vi "20210415_01_ATA_FPGA.vi"() -> ()   [LabVIEW 2018]
doc: "This FPGA VI transfers data samples to the host using a stream. The stream is controlled from the host."
uses:
  <vilib>/Platform/TimedLoop/XDataNode/wakeup.ctl
  <vilib>/Platform/TimedLoop/XDataNode/XDNodeRunTimeDep.lvlib
  <vilib>/Platform/TimedLoop/XDataNode/nitl_modes.ctl
  <vilib>/Platform/TimedLoop/XDataNode/timing_clust.ctl
  <vilib>/Platform/TimedLoop/XDataNode/XDataNode.xnode
  <vilib>/eio/EIONode/EIONode.xnode
  <vilib>/rvi/eio/common/nirviEmuTemplateMethod_errors.vi
  <vilib>/rvi/DataTransferAndStorage/Container/XNode/niFpgaContainer.xnode
  <instrlib>/_niInstr/Basic Elements/v1/FPGA/niInstr Basic Elements v1 FPGA.lvlib
  <vilib>/rvi/FXPMathLib/FxpInterpret/XNode/nifxpmath_Interpret.xnode
  <vilib>/rvi/FXPMathLib/FxpMul/XNode/nifxpmath_Multiplier.xnode
  <vilib>/rvi/FXPMathLib/sim/FxpSim.dll
  <vilib>/rvi/FXPMathLib/FxpAdd/XNode/nifxpmath_Add.xnode
  <vilib>/rvi/Analysis/measure/FFT/XNode/niFpgaFFT.xnode
  <instrlib>/_niInstr/Basic Elements/v1/FPGA/Private/Count Up U32.vi
  <vilib>/rvi/Memory/Memory_Emulation/niFpgaMemoryEmulationRefIn.vi
  <vilib>/fxp/LVFixedPointQuantizationPolicyTypeDef.ctl
  <vilib>/rvi/Analysis/measure/FFT/simModelSupport/niFpgaFFTSimDfxp.ctl
  <vilib>/rvi/Analysis/measure/FFT/simModelSupport/niFpgaFFTSimArithmeticProperties.ctl
  <vilib>/rvi/Analysis/measure/FFT/simModelSupport/niFPGA FFT Sim Types.ctl
  <vilib>/rvi/Analysis/measure/FFT/simModelSupport/niFPGA FFT Outside SCTL Sim Properties.ctl
  <vilib>/rvi/Analysis/measure/FFT/simModelSupport/niFpgaFFTSimModelOutsideSCTLCore.vi
  <vilib>/rvi/LocalResourceManager/LocalResourceManager.xnode
  <vilib>/rvi/DataTransferAndStorage/Container/Common/niFpgaContainerGetUniqueNameForEmu.vi
  <vilib>/rvi/DataTransferAndStorage/Container/Common/niFpgaContainerSetEmuInfo.vi
  <vilib>/rvi/eio/common/nirviEmuReportErrorAndStop.vi
  <vilib>/rvi/FIFO/Fifo_Resource/niFpgaFifoEmulationRefIn.vi
  <vilib>/rvi/FIFO/Fifo_Resource/nirvififoEmulationRead.vi
  <vilib>/rvi/interface/RandomDataEmulation/nirviRandomDataFpgaMultiElementTemplate.vi
  <instrlib>/_niInstr/Basic Elements/v1/FPGA/Private/Count Up U16.vi
  FPGA_Controls/FilterStageEnum.ctl
  FPGA_Controls/FPGA_Enable_Clust.ctl
  FPGA_Controls/FPGA_Shift_Enable.ctl
  <instrlib>/_niInstr/Basic Elements/v1/FPGA/Private/Count Up U8.vi
  FPGA_Controls/FPGA_Scale_Clust.ctl
  FPGA_Controls/FPGA_Probe_Clust.ctl
panel:
  out "5_Seconds_Elapsed":bool
  out "Write to FIFO 2":bool
  out "Write to FIFO":bool
  in  "EnableFIFO":bool
  out "AI0_Unshifted_Index":u32
  out "AI0_Co_Beac_Q_Index":fxp<+/-,24,1>
  out "AI0_Co_I_Index":fxp<+/-,24,1>
  out "MaxMeas":fxp<+/-,24,1>
  in  "Ramp?":bool
  out "AI1_Over":bool
  out "AI0_Over":bool
  in  "Simulate?":bool
  out "Chan1_Beac_QProbe":T1
  out "Chan1_Beac_IProbe":T1
  out "Chan1_Cal_QProbe":T1
  out "Chan0_Beac_QProbe":T1
  out "Chan0_Beac_IProbe":T1
  out "Chan0_Cal_QProbe":T1
  out "NoiseFloorFFT_LoopCount 2":i32
  out "ReceiverTimed Out 2":bool
  out "SuccessiveIndeces 2":u16[](array[numeric])
  in  "#Avg 2":u16=1
  in  "ScaleMeasurement 2":fxp<+/-,16,1>
  in  "Scale_Step1_2":fxp<+/-,17,17>
  in  "EnableStep1_2":bool
  out "Probe 2_2":fxp<+/-,16,16>
  out "Probe 3_2":fxp<+/-,16,1>
  out "Probe 5_2":fxp<+/-,16,2>
  out "Probe 7_2":fxp<+/-,18,1>
  in  "Scale_NoiseFloor 2":fxp<+/-,30,30>
  out "Probe 21_2":fxp<+/-,24,5>
  out "Probe 22_2":fxp<+/-,54,35>
  out "Probe 23_2":fxp<+/-,54,1>
  out "Probe 24_2":fxp<+/-,16,1>
  in  "Offset 2":fxp<+/-,16,16>
  in  "Scale 2":T2={"Scale_Step4"=1.0, "Scale_Step5"=1.0, "Scale_Step6"=1.0, "Scale_Step7"=1.0}
  in  "Enable 2":T3
  in  "FreqShiftCal 2":fxp<+/-,48,0> format="%#.48g"
  out "Chan1_Cal_IProbe":T1
  in  "FreqShiftBeac 2":fxp<+/-,48,0> format="%#.48g"
  out "NoiseFloorFIFOTimeOut 2":bool
  out "Sends 2":u32
  in  "SampleCountReset 2":u32=125000000
  out "Probe 1_2":i16
  out "Probe Offsetd 2":fxp<+/-,16,16>
  out "Probe Offsetd":fxp<+/-,16,16>
  in  "Sample Clock Commit":bool
  in  "Sample Clock Select":u8
  out "SPI Idle":bool
  out "Configuration Error":bool
  out "Synthesizer Locked":bool
  out "Probe 1":i16
  in  "#Avg":u16=1
  in  "SampleCountReset":u32=125000000
  out "ReceiverTimed Out":bool
  out "Sends":u32
  out "SuccessiveIndeces":u16[](array[numeric])
  out "NoiseFloorFFT_LoopCount":i32
  out "NoiseFloorFIFOTimeOut":bool
  in  "FreqShiftBeac":fxp<+/-,48,0> format="%#.48g"
  out "AI0_Cal_IProbe":T1
  in  "Scale":T2={"Scale_Step4"=1.0, "Scale_Step5"=1.0, "Scale_Step6"=1.0, "Scale_Step7"=1.0}
  in  "Enable":T3
  in  "Offset":fxp<+/-,16,16>
  out "Probe 24":fxp<+/-,16,1>
  out "Probe 23":fxp<+/-,54,1>
  out "Probe 22":fxp<+/-,54,35>
  out "Probe 21":fxp<+/-,24,5>
  in  "Scale_NoiseFloor":fxp<+/-,30,30>
  out "Probe 7":fxp<+/-,18,1>
  out "Probe 5":fxp<+/-,16,2>
  out "Probe 3":fxp<+/-,16,1>
  out "Probe 2":fxp<+/-,16,16>
  in  "EnableStep1":bool
  in  "Scale_Step1":fxp<+/-,17,17>
  in  "ScaleMeasurement":fxp<+/-,16,1>
  in  "FreqShiftCal":fxp<+/-,48,0> format="%#.48g"
  out "IO Module\\Initialization Done":bool
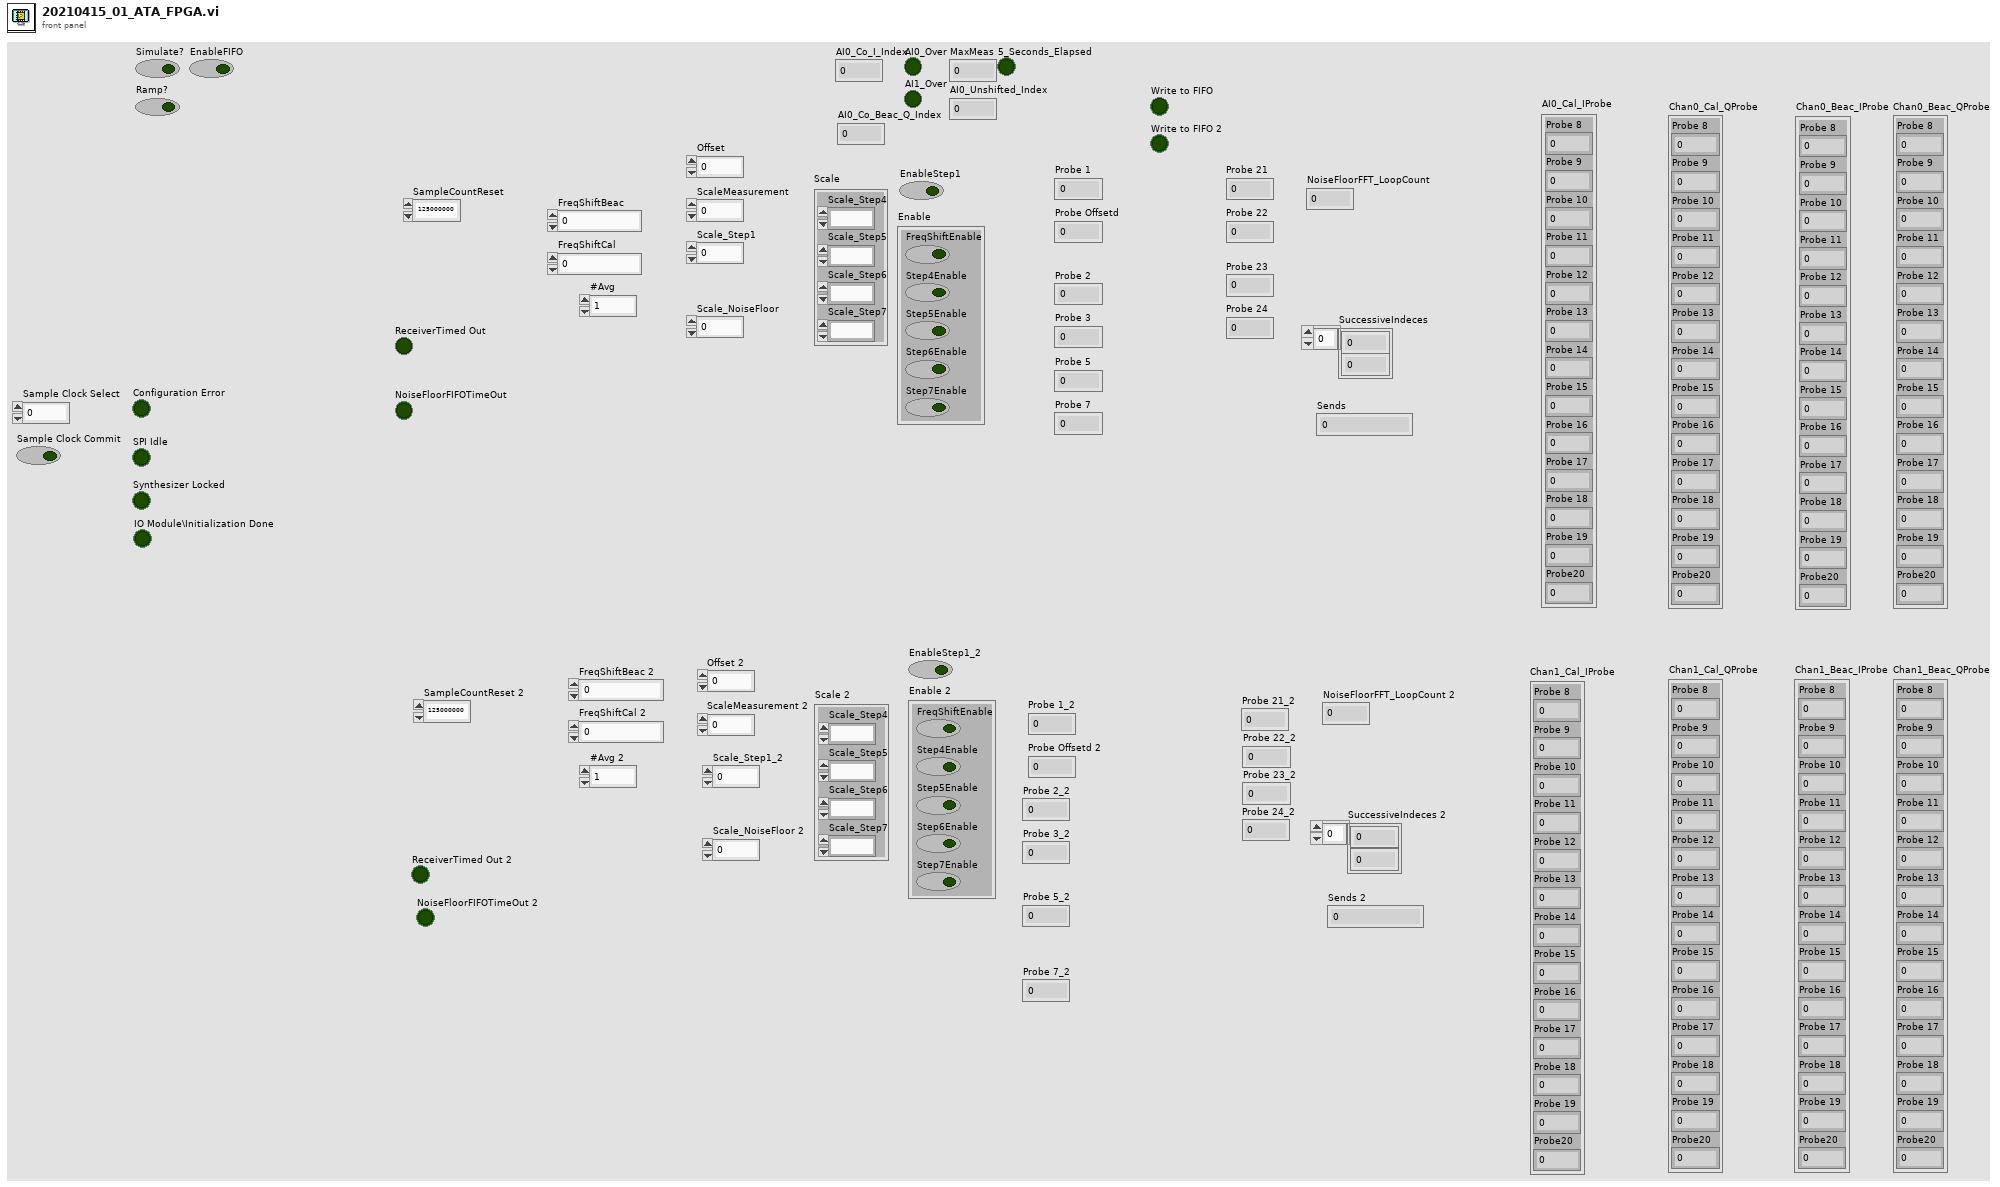
[diagram p1: front panel]
types:
  T1 = typedef "FPGA_Probe_Clust.ctl" = cluster{"Probe 8":fxp<+/-,18,1>, "Probe 9":fxp<+/-,24,1>, "Probe 10":fxp<+/-,24,1>, "Probe 11":fxp<+/-,24,1>, "Probe 12":fxp<+/-,47,24>, "Probe 13":fxp<+/-,24,1>, "Probe 14":fxp<+/-,25,2>, "Probe 15":fxp<+/-,48,25>, "Probe 16":fxp<+/-,24,1>, "Probe 17":fxp<+/-,25,2>, "Probe 18":fxp<+/-,48,25>, "Probe 19":fxp<+/-,24,1>, "Probe20":fxp<+/-,24,1>}
  T2 = typedef "FPGA_Scale_Clust.ctl" = cluster{"Scale_Step4":fxp<+/-,23,23>, "Scale_Step5":fxp<+/-,23,23>, "Scale_Step6":fxp<+/-,23,23>, "Scale_Step7":fxp<+/-,23,23>}
  T3 = typedef "FPGA_Enable_Clust.ctl" = cluster{"FreqShiftEnable":bool, "Step4Enable":bool, "Step5Enable":bool, "Step6Enable":bool, "Step7Enable":bool}
  T4 = typedef "XDNodeRunTimeDep.lvlib/timing_clust.ctl" = cluster{"Expected End [f-1]":u64, "Actual End [f-1]":u64, "Finished Late? [f-1]":bool, "Expected End [i-1]":u64, "Actual End [i-1]":u64, "Finished Late? [i-1]":bool, "Expected Start [i]":u64, "Actual Start [i]":u64, "Expected Start [f]":u64, "Actual Start [f]":u64, "Source Name":string, "Structure Name":string, "Period":i64, "Deadline":i64, "Offset":i64, "Start":i64, "Priority":i32, "Timeout":i32, "Mode":T5, "Wakeup Reason":T6, "Error":errorcluster, "Source Type":string, "Secondary Source Type":string, "Global End Time":u64, "Global Start Time":u64, "Frame Duration":u64, "Iteration Duration":u64, "Assigned CPU":i32, "I/O Scan Engine Mode":u32}
  T5 = typedef "XDNodeRunTimeDep.lvlib/nitl_modes.ctl" = enum32{"No Change", "Process missed periods, maintain original phase", "Discard missed periods, maintain original phase", "Process missed periods, ignore original phase", "Discard missed periods, ignore original phase"}
  T6 = typedef "XDNodeRunTimeDep.lvlib/wakeup.ctl" = enum32{"Normal", "Aborted", "Asynchronous wakeup", "Timing source error", "Timed loop error", "Timeout"}
  T7 = typedef "FPGA_Shift_Enable.ctl" = cluster{"EnableFIFO":bool, "EnableStages":T3}
  T8 = typedef "FilterStageEnum.ctl" = enum16{"Digitiz0", "Digitiz1", "ScaleMeas", "Scale1", "Scale4", "Scale5", "Scale6", "Scale7"}
  T9 = typedef "FPGA_ShiftOutput.ctl" = cluster{"Index":fxp<+/-,24,1>, "output valid":bool, "Data out":fxp<+/-,24,1>, "Probe":T1}
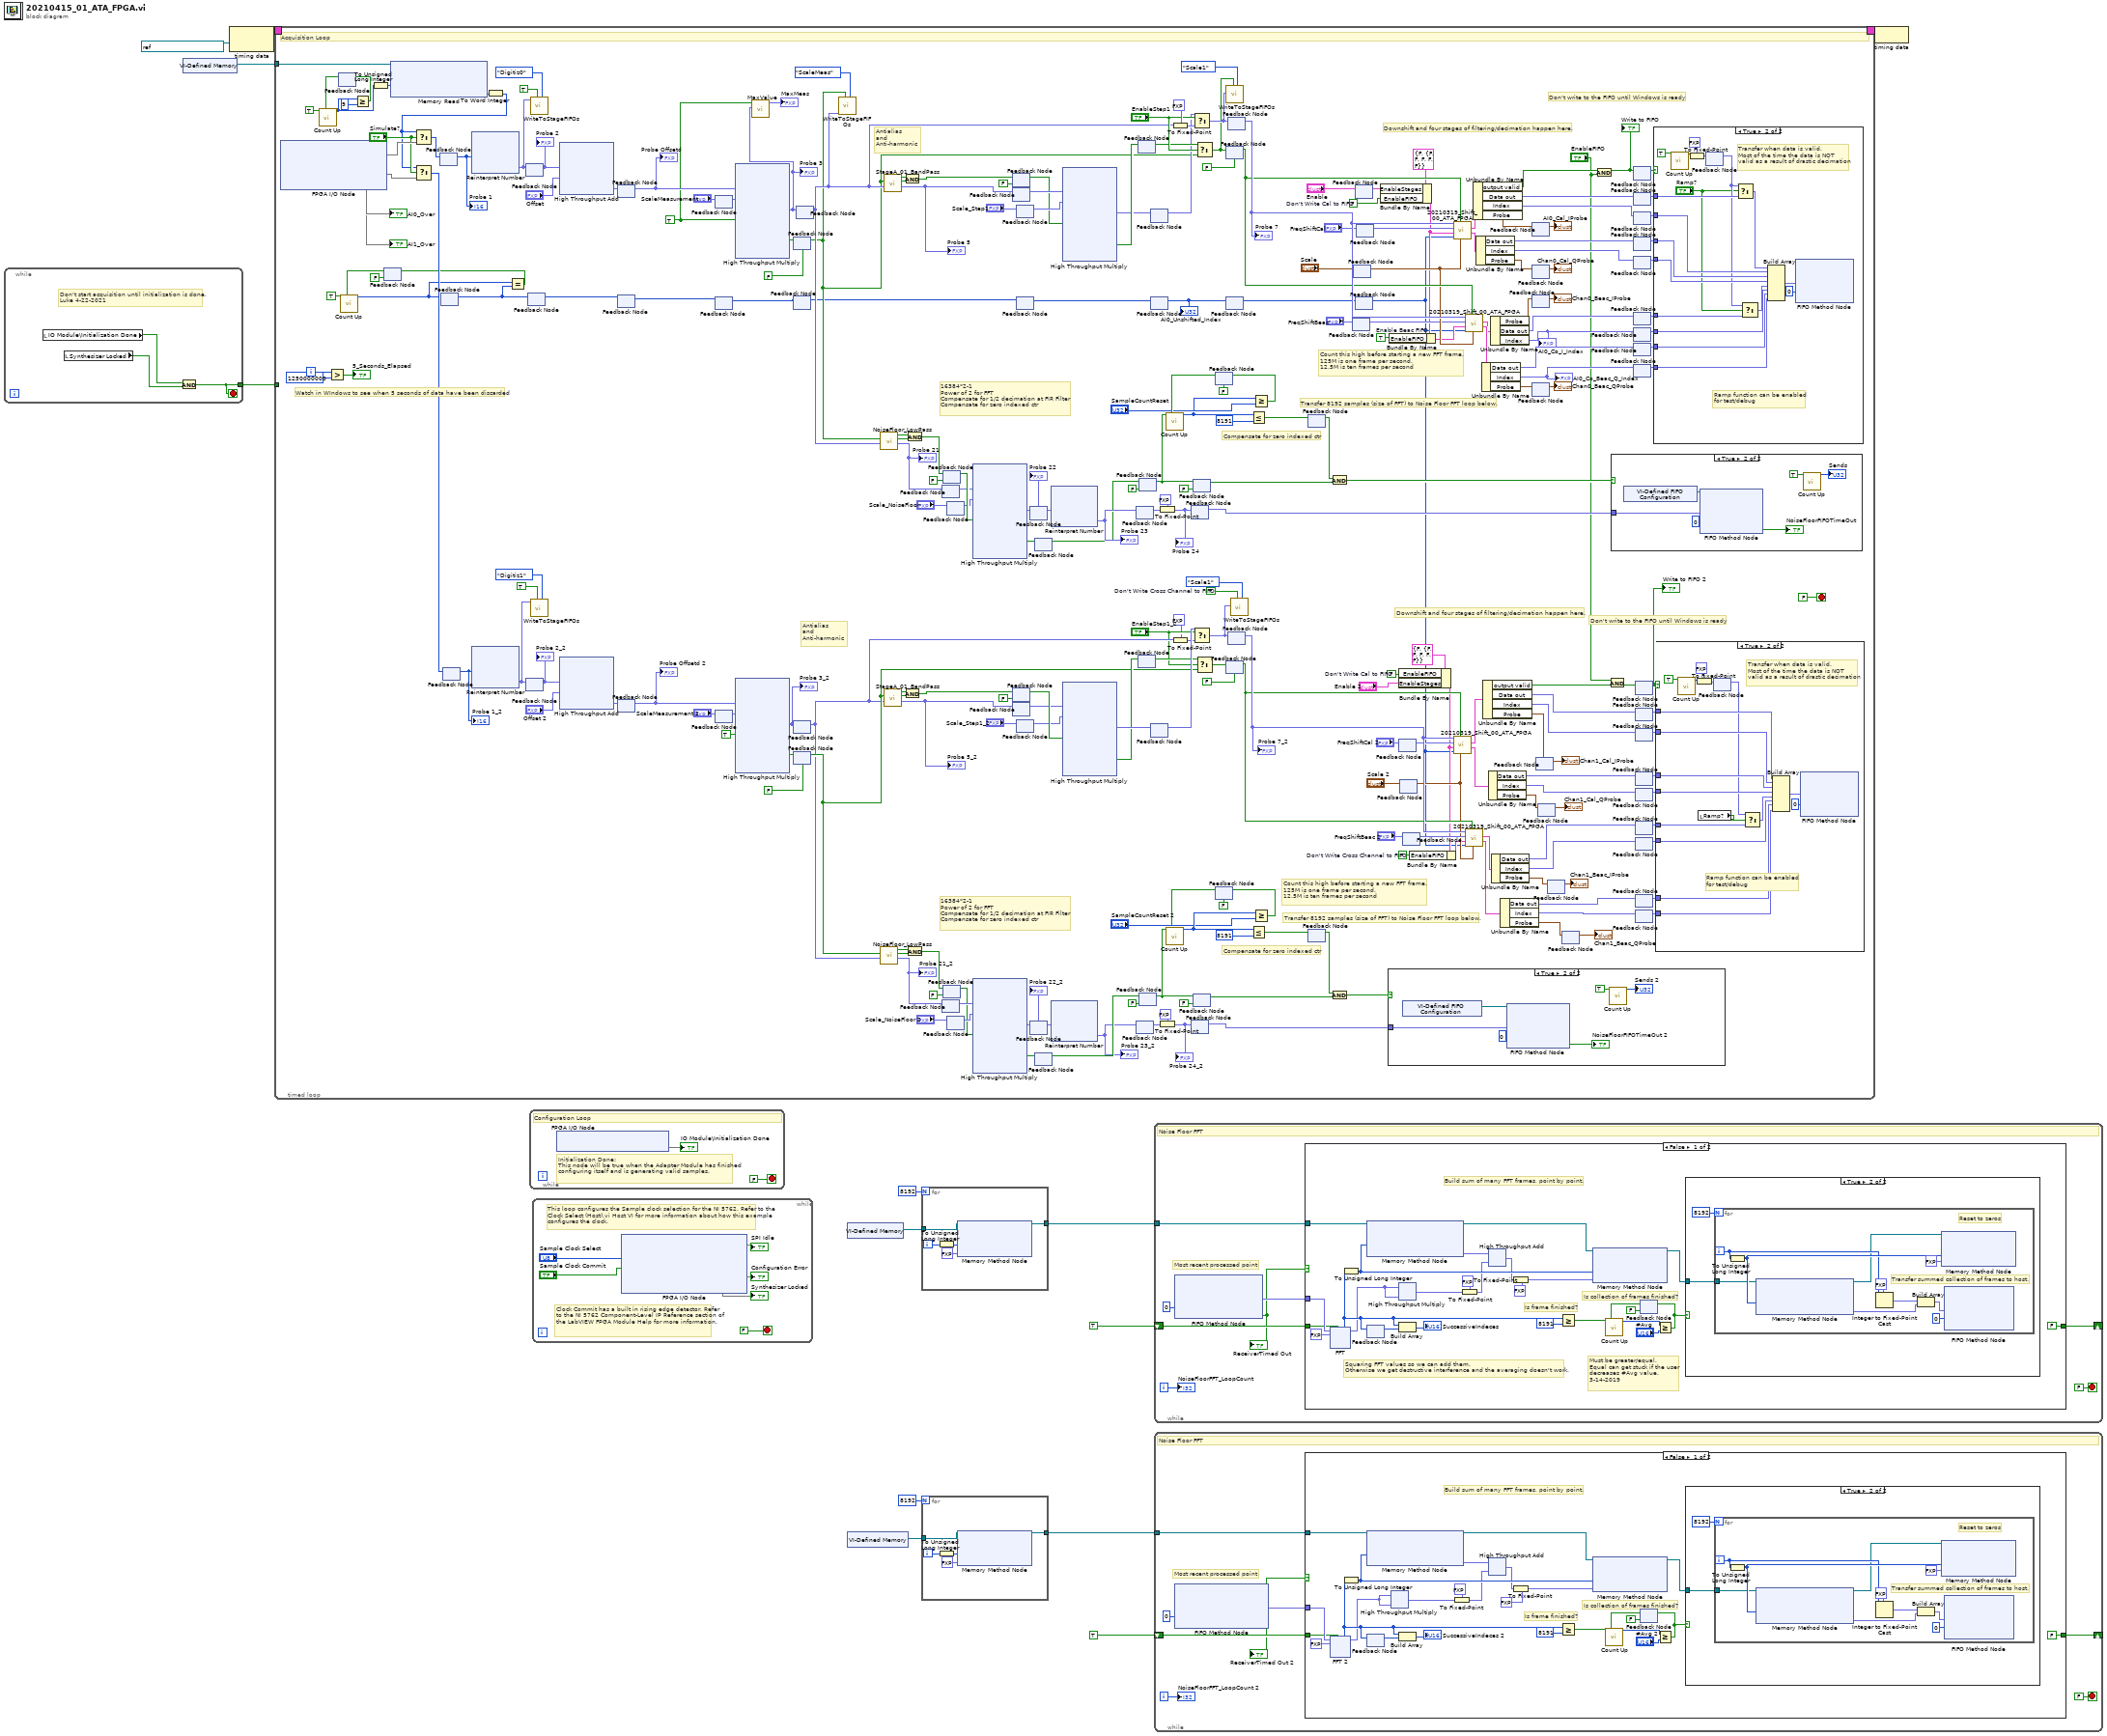
[diagram p0: block diagram]
diagram:
  n1 = while {
    tunnel: [w14] -> w1
    stop <- w14 stop-if-true
    # "Don't start acquisition until initialization is done.\nLuke 4-22-2021"
    n2 = local read "IO Module\\Initialization Done"() -> (w16:bool)
    n3 = local read "Synthesizer Locked"() -> (w15:bool)
    n4 = And(x=w16, y=w15) -> (x .and. y?=w14:bool)
  }
  n5 = xnode "VI-Defined Memory"() -> ("Memory Out"=w2:refnum<k21>)
  n6 = node-c288(refnum<k21> "IO Module\\Data Clock" ("Source Name")) -> (w13:T4)
  n7 = timed-loop {
    timing: w13 -> [_]
    timing-out: [_] -> w12
    tunnel: w2 -> [w118]
    tunnel: w1 -> [_]
    i -> [w19]
    stop <- FALSE stop-if-true
    w66 = FALSE  # Don't Write Cal to FIFO
    w63 = TRUE  # Enable Beac FIFO
    w94 = FALSE  # Don't Write Cross Channel to FIFO
    w52 = FALSE  # Don't Write Cross Channel to FIFO
    w58 = FALSE  # Don't Write Cal to FIFO
    w107 = TRUE ("input valid")
    # "Watch in WIndows to see when 5 seconds of data have been discarded"
    # "Don't write to the FIFO until Windows is ready"
    # "Don't write to the FIFO until Windows is ready"
    # "Downshift and four stages of filtering/decimation happen here."
    # "Downshift and four stages of filtering/decimation happen here."
    # "Antialias\nand\nAnti-harmonic"
    # "Compensate for zero indexed ctr"
    # "16384*2-1\nPower of 2 for FFT\nCompensate for 1/2 decimation at FIR Filter\nCompensate for zero indexed ctr"
    # "Transfer 8192 samples (size of FFT) to Noise Floor FFT loop below."
    # "Count this high before starting a new FFT frame.\n125M is one frame per second.\n12.5M is ten frames per second"
    # "Antialias\nand\nAnti-harmonic"
    # "Compensate for zero indexed ctr"
    # "16384*2-1\nPower of 2 for FFT\nCompensate for 1/2 decimation at FIR Filter\nCompensate for zero indexed ctr"
    # "Transfer 8192 samples (size of FFT) to Noise Floor FFT loop below."
    # "Count this high before starting a new FFT frame.\n125M is one frame per second.\n12.5M is ten frames per second"
    # "Acquisition Loop"
    n8 = xnode "FPGA I/O Node"() -> ("IO Module\\AI 0 Data"=w117, "IO Module\\AI 0 Over Range"=→"AI0_Over", "IO Module\\AI 1 Data"=w112, "IO Module\\AI 1 Over Range"=→"AI1_Over")  [unwired: 4 in, 4 out]
    n9 = Greater?(x=w19, y=1250000000) -> (0:→"5_Seconds_Elapsed":bool)
    n10 = feedback #1() -> (w119:bool)  [unwired: 1 in]
    n11 = call-poly <instrlib>:"Count Up.vi"("increment"=TRUE, "reset"=w119) -> ("count out"=w122:u8)  [unwired: 13 in]
    n12 = Greater Or Equal?(x=w122, y=u8 9) -> (x >= y?=w120:bool)
    n13 = feedback-in #1(w120) -> ()
    n14 = To Unsigned Long Integer(number=w122) -> (unsigned 32bit integer=w124:u32)
    n15 = feedback #2(FALSE) -> (w28:bool)
    n16 = call-poly <instrlib>:"Count Up.vi"("increment"=TRUE, "reset"=w28) -> ("count out"=w26:u32)  [unwired: 13 in]
    n17 = xnode ("Memory Read")("Address"=w124, "Memory In"=w118) -> ("Data"=w115:i8)  [unwired: 1 out]
    n18 = feedback #3() -> (w226:i16)  [unwired: 1 in]
    "Probe 1" <- w226
    n19 = feedback #4() -> (w25:u32)  [unwired: 1 in]
    n20 = feedback-in #4(w26) -> ()
    n21 = feedback #5() -> (w207:i16)  [unwired: 1 in]
    "Probe 1_2" <- w207
    n22 = xnode "Reinterpret Number"("x"=w226) -> ("y"=w98:fxp<+/-,16,16>)
    n23 = xnode "Reinterpret Number"("x"=w207) -> ("y"=w97:fxp<+/-,16,16>)
    n24 = To Word Integer(number=w115) -> (16bit integer=w111:i16)
    n25 = Select(t=w111, s="Simulate?", f=w117) -> (s? t:f=w116:i16)
    n26 = Select(t=w111, s="Simulate?", f=w112) -> (s? t:f=w113:i16)
    n27 = feedback-in #3(w116) -> ()
    n28 = feedback-in #5(w113) -> ()
    n29 = Equal?(x=w26, y=w25) -> (x = y?=w29:bool)
    n30 = feedback-in #2(w29) -> ()
    n31 = feedback #6() -> (w239:fxp<+/-,16,16>)  [unwired: 1 in]
    "Probe 2" <- w239
    n32 = feedback-in #6(w98) -> ()
    n33 = feedback #7() -> (w198:fxp<+/-,16,16>)  [unwired: 1 in]
    "Probe 2_2" <- w198
    n34 = feedback-in #7(w97) -> ()
    n35 = feedback #8() -> (w30:u32)  [unwired: 1 in]
    n36 = feedback-in #8(w25) -> ()
    n37 = call "WriteToStageFIFOs.vi"("Stage"=FilterStageEnum."Digitiz0", "Enable"=TRUE, "Digitiz"=w98) -> ()  [unwired: 9 in]
    n38 = call "WriteToStageFIFOs.vi"("Stage"=FilterStageEnum."Digitiz1", "Enable"=TRUE, "Digitiz"=w97) -> ()  [unwired: 9 in]
    n39 = xnode ("High Throughput Add")("x"=w239, "y"="Offset") -> ("x+y"=w238:fxp<+/-,16,16>)
    n40 = xnode ("High Throughput Add")("x"=w198, "y"="Offset 2") -> ("x+y"=w100:fxp<+/-,16,16>)
    n41 = feedback #9() -> (w108:fxp<+/-,16,16>)  [unwired: 1 in]
    "Probe Offsetd" <- w108
    n42 = feedback-in #9(w238) -> ()
    n43 = feedback #10() -> (w87:u32)  [unwired: 1 in]
    n44 = feedback-in #10(w30) -> ()
    n45 = feedback #11() -> (w99:fxp<+/-,16,16>)  [unwired: 1 in]
    "Probe Offsetd 2" <- w99
    n46 = feedback-in #11(w100) -> ()
    n47 = feedback #12() -> (w267:fxp<+/-,16,1>)  [unwired: 1 in]
    n48 = feedback-in #12("ScaleMeasurement") -> ()
    n49 = feedback #13() -> (w86:u32)  [unwired: 1 in]
    n50 = feedback-in #13(w87) -> ()
    n51 = feedback #14() -> (w168:fxp<+/-,16,1>)  [unwired: 1 in]
    n52 = feedback-in #14("ScaleMeasurement 2") -> ()
    n53 = xnode ("High Throughput Multiply")("x"=w108, "y"=w267, "input valid"=w107) -> ("x*y"=w106:fxp<+/-,16,1>, "output valid"=w241:bool)  [unwired: 1 in, 1 out]
    "Probe 3" <- w106
    n54 = xnode ("High Throughput Multiply")("x"=w99, "y"=w168, "input valid"=TRUE) -> ("x*y"=w165:fxp<+/-,16,1>, "output valid"=w196:bool)  [unwired: 1 in, 1 out]
    "Probe 3_2" <- w165
    n55 = call "MaxValue.vi"("NewValue"=w106, "DataValid"=w107) -> ("Max"=→"MaxMeas":fxp<+/-,24,1>)  [unwired: 9 in]
    n56 = feedback #15(FALSE ("output valid")) -> (w89:bool)
    n57 = feedback-in #15(w241) -> ()
    n58 = feedback #16() -> (w85:u32)  [unwired: 1 in]
    n59 = feedback-in #16(w86) -> ()
    n60 = feedback #17() -> (w210:fxp<+/-,16,1>)  [unwired: 1 in]
    n61 = feedback-in #17(w165) -> ()
    n62 = feedback #18(FALSE ("output valid")) -> (w212:bool)
    n63 = feedback-in #18(w196) -> ()
    n64 = feedback #19() -> (w90:fxp<+/-,16,1>)  [unwired: 1 in]
    n65 = feedback-in #19(w106) -> ()
    n66 = call "WriteToStageFIFOs.vi"("Stage"=FilterStageEnum."ScaleMeas", "Enable"=w89, "ScaleMeas"=w90) -> ()  [unwired: 9 in]
    n67 = call "NoiseFloor_LowPass.vi"("s_axis_data_tdata"=w90, "s_axis_data_tvalid"=w89) -> ("m_axis_data_tdata"=w251:fxp<+/-,24,5>, "m_axis_data_tvalid"=w258:bool, "s_axis_data_tready"=w259:bool)  [unwired: 7 in]
    "Probe 21" <- w251
    n68 = call "NoiseFloor_LowPass.vi"("s_axis_data_tdata"=w210, "s_axis_data_tvalid"=w212) -> ("m_axis_data_tdata"=w186:fxp<+/-,24,5>, "m_axis_data_tvalid"=w179:bool, "s_axis_data_tready"=w178:bool)  [unwired: 7 in]
    "Probe 21_2" <- w186
    n69 = call "StageA_01_BandPass.vi"("s_axis_data_tdata"=w90, "s_axis_data_tvalid"=w89) -> ("m_axis_data_tdata"=w223:fxp<+/-,16,2>, "m_axis_data_tvalid"=w272:bool, "s_axis_data_tready"=w273:bool)  [unwired: 7 in]
    "Probe 5" <- w223
    n70 = call "StageA_01_BandPass.vi"("s_axis_data_tdata"=w210, "s_axis_data_tvalid"=w212) -> ("m_axis_data_tdata"=w211:fxp<+/-,16,2>, "m_axis_data_tvalid"=w162:bool, "s_axis_data_tready"=w161:bool)  [unwired: 7 in]
    "Probe 5_2" <- w211
    n71 = And(x=w273, y=w272) -> (x .and. y?=w224:bool)
    n72 = And(x=w161, y=w162) -> (x .and. y?=w209:bool)
    n73 = And(x=w259, y=w258) -> (x .and. y?=w250:bool)
    n74 = And(x=w178, y=w179) -> (x .and. y?=w187:bool)
    n75 = feedback #20() -> (w252:fxp<+/-,24,5>)  [unwired: 1 in]
    n76 = feedback-in #20(w251) -> ()
    n77 = feedback #21() -> (w185:fxp<+/-,24,5>)  [unwired: 1 in]
    n78 = feedback-in #21(w186) -> ()
    n79 = feedback #22(FALSE ("s_axis_data_tvalid")) -> (w255:bool)
    n80 = feedback-in #22(w250) -> ()
    n81 = feedback #23(FALSE ("s_axis_data_tvalid")) -> (w182:bool)
    n82 = feedback-in #23(w187) -> ()
    n83 = feedback #24() -> (w254:fxp<+/-,30,30>)  [unwired: 1 in]
    n84 = feedback-in #24("Scale_NoiseFloor") -> ()
    n85 = feedback #25() -> (w183:fxp<+/-,30,30>)  [unwired: 1 in]
    n86 = feedback-in #25("Scale_NoiseFloor 2") -> ()
    n87 = xnode ("High Throughput Multiply")("x"=w252, "y"=w254, "input valid"=w255) -> ("x*y"=w247:fxp<+/-,54,35>, "output valid"=w244:bool)  [unwired: 1 in, 1 out]
    "Probe 22" <- w247
    n88 = xnode ("High Throughput Multiply")("x"=w185, "y"=w183, "input valid"=w182) -> ("x*y"=w190:fxp<+/-,54,35>, "output valid"=w193:bool)  [unwired: 1 in, 1 out]
    "Probe 22_2" <- w190
    n89 = feedback #26() -> (w269:fxp<+/-,16,2>)  [unwired: 1 in]
    n90 = feedback-in #26(w223) -> ()
    n91 = feedback #27() -> (w166:fxp<+/-,16,2>)  [unwired: 1 in]
    n92 = feedback-in #27(w211) -> ()
    n93 = feedback #28(FALSE ("s_axis_data_tvalid")) -> (w265:bool)
    n94 = feedback-in #28(w224) -> ()
    n95 = feedback #29(FALSE ("s_axis_data_tvalid")) -> (w170:bool)
    n96 = feedback-in #29(w209) -> ()
    n97 = feedback #30() -> (w266:fxp<+/-,17,17>)  [unwired: 1 in]
    n98 = feedback-in #30("Scale_Step1") -> ()
    n99 = feedback #31() -> (w84:u32)  [unwired: 1 in]
    n100 = feedback-in #31(w85) -> ()
    n101 = feedback #32() -> (w169:fxp<+/-,17,17>)  [unwired: 1 in]
    n102 = feedback-in #32("Scale_Step1_2") -> ()
    n103 = feedback #33() -> (w246:fxp<+/-,54,35>)  [unwired: 1 in]
    n104 = feedback-in #33(w247) -> ()
    n105 = feedback #34() -> (w191:fxp<+/-,54,35>)  [unwired: 1 in]
    n106 = feedback-in #34(w190) -> ()
    n107 = feedback #35() -> (w243:bool)  [unwired: 1 in]
    n108 = feedback-in #35(w244) -> ()
    n109 = feedback #36() -> (w194:bool)  [unwired: 1 in]
    n110 = feedback-in #36(w193) -> ()
    n111 = xnode "Reinterpret Number"("x"=w246) -> ("y"=w245:fxp<+/-,54,1>)
    "Probe 23" <- w245
    n112 = xnode "Reinterpret Number"("x"=w191) -> ("y"=w192:fxp<+/-,54,1>)
    "Probe 23_2" <- w192
    n113 = xnode ("High Throughput Multiply")("x"=w269, "y"=w266, "input valid"=w265) -> ("x*y"=w220:fxp<+/-,18,1>, "output valid"=w222:bool)  [unwired: 1 in, 1 out]
    n114 = xnode ("High Throughput Multiply")("x"=w166, "y"=w169, "input valid"=w170) -> ("x*y"=w215:fxp<+/-,18,1>, "output valid"=w213:bool)  [unwired: 1 in, 1 out]
    n115 = feedback #37() -> (w248:fxp<+/-,54,1>)  [unwired: 1 in]
    n116 = feedback-in #37(w245) -> ()
    n117 = feedback #38() -> (w189:fxp<+/-,54,1>)  [unwired: 1 in]
    n118 = feedback-in #38(w192) -> ()
    n119 = feedback #39() -> (w221:bool)  [unwired: 1 in]
    n120 = feedback-in #39(w222) -> ()
    n121 = feedback #40() -> (w214:bool)  [unwired: 1 in]
    n122 = feedback-in #40(w213) -> ()
    n123 = feedback #41(FALSE ("output valid")) -> (w237:bool)
    n124 = feedback-in #41(w243) -> ()
    n125 = feedback #42(FALSE ("output valid")) -> (w199:bool)
    n126 = feedback-in #42(w194) -> ()
    n127 = feedback #43() -> (w219:fxp<+/-,18,1>)  [unwired: 1 in]
    n128 = feedback-in #43(w220) -> ()
    n129 = feedback #44() -> (w83:u32)  [unwired: 1 in]
    "AI0_Unshifted_Index" <- w83
    n130 = feedback-in #44(w84) -> ()
    n131 = feedback #45() -> (w216:fxp<+/-,18,1>)  [unwired: 1 in]
    n132 = feedback-in #45(w215) -> ()
    n133 = To Fixed-Point(fixed-point type=fxp<+/-,16,1> 0.0, number=w248) -> (fixed-point=w227:fxp<+/-,16,1>)
    "Probe 24" <- w227
    n134 = To Fixed-Point(fixed-point type=fxp<+/-,16,1> 0.0, number=w189) -> (fixed-point=w206:fxp<+/-,16,1>)
    "Probe 24_2" <- w206
    n135 = To Fixed-Point(fixed-point type=fxp<+/-,18,1> 0.0, number=w90) -> (fixed-point=w263:fxp<+/-,18,1>)
    n136 = To Fixed-Point(fixed-point type=fxp<+/-,18,1> 0.0, number=w210) -> (fixed-point=w173:fxp<+/-,18,1>)
    n137 = feedback #46() -> (w228:fxp<+/-,16,1>)  [unwired: 1 in]
    n138 = feedback-in #46(w227) -> ()
    n139 = feedback #47() -> (w205:fxp<+/-,16,1>)  [unwired: 1 in]
    n140 = feedback-in #47(w206) -> ()
    n141 = feedback #48(FALSE ("output valid")) -> (w235:bool)
    n142 = feedback-in #48(w237) -> ()
    n143 = feedback #49(FALSE ("output valid")) -> (w201:bool)
    n144 = feedback-in #49(w199) -> ()
    n145 = Select(t=w219, s="EnableStep1", f=w263) -> (s? t:f=w102:fxp<+/-,18,1>)
    n146 = Select(t=w216, s="EnableStep1_2", f=w173) -> (s? t:f=w95:fxp<+/-,18,1>)
    n147 = Select(t=w221, s="EnableStep1", f=w89) -> (s? t:f=w88:bool)
    n148 = Select(t=w214, s="EnableStep1_2", f=w212) -> (s? t:f=w171:bool)
    n149 = feedback #50(FALSE ("reset")) -> (w278:bool)
    n150 = call-poly <instrlib>:"Count Up.vi"("increment"=w237, "reset"=w278) -> ("count out"=w271:u32)  [unwired: 13 in]
    n151 = feedback #51(FALSE ("reset")) -> (w156:bool)
    n152 = call-poly <instrlib>:"Count Up.vi"("increment"=w199, "reset"=w156) -> ("count out"=w163:u32)  [unwired: 13 in]
    n153 = feedback #52(FALSE ("s_axis_data_tvalid")) -> (w154:bool)
    n154 = feedback-in #52(w88) -> ()
    n155 = feedback #53() -> (w82:u32)  [unwired: 1 in]
    n156 = feedback-in #53(w83) -> ()
    n157 = feedback #54(FALSE ("s_axis_data_tvalid")) -> (w148:bool)
    n158 = feedback-in #54(w171) -> ()
    n159 = call "WriteToStageFIFOs.vi"("Stage"=FilterStageEnum."Scale1", "Enable"=w88, "Scale1"=w102) -> ()  [unwired: 9 in]
    n160 = feedback #55() -> (w218:fxp<+/-,18,1>)  [unwired: 1 in]
    "Probe 7" <- w218
    n161 = feedback-in #55(w102) -> ()
    n162 = feedback #56() -> (w217:fxp<+/-,18,1>)  [unwired: 1 in]
    "Probe 7_2" <- w217
    n163 = feedback-in #56(w95) -> ()
    n164 = call "WriteToStageFIFOs.vi"("Stage"=FilterStageEnum."Scale1", "Enable"=w94, "Scale1"=w95) -> ()  [unwired: 9 in]
    n165 = Less Or Equal?(x=w271, y=u32 8191) -> (x <= y?=w279:bool)
    n166 = Less Or Equal?(x=w163, y=u32 8191) -> (x <= y?=w155:bool)
    n167 = Greater Or Equal?(x=w271, y="SampleCountReset") -> (x >= y?=w275:bool)
    n168 = feedback-in #50(w275) -> ()
    n169 = Greater Or Equal?(x=w163, y="SampleCountReset 2") -> (x >= y?=w159:bool)
    n170 = feedback-in #51(w159) -> ()
    n171 = feedback #57() -> (w236:bool)  [unwired: 1 in]
    n172 = feedback-in #57(w279) -> ()
    n173 = feedback #58() -> (w200:bool)  [unwired: 1 in]
    n174 = feedback-in #58(w155) -> ()
    n175 = And(x=w236, y=w235) -> (x .and. y?=w234:bool)
    n176 = And(x=w200, y=w201) -> (x .and. y?=w202:bool)
    n177 = feedback #59() -> (w137:fxp<+/-,48,0>)  [unwired: 1 in]
    n178 = feedback-in #59("FreqShiftBeac") -> ()
    n179 = feedback #60() -> (w139:T2)  [unwired: 1 in]
    n180 = feedback-in #60("Scale") -> ()
    n181 = feedback #61() -> (w67:T3)  [unwired: 1 in]
    n182 = feedback-in #61("Enable") -> ()
    n183 = feedback #62() -> (w24:u32)  [unwired: 1 in]
    n184 = feedback-in #62(w82) -> ()
    n185 = feedback #63() -> (w135:fxp<+/-,48,0>)  [unwired: 1 in]
    n186 = feedback-in #63("FreqShiftCal") -> ()
    n187 = Bundle By Name(cluster=T7 {"EnableFIFO"=FALSE, "EnableStages"={"FreqShiftEnable"=FALSE, "Step4Enable"=FALSE, "Step5Enable"=FALSE, "Step6Enable"=FALSE, "Step7Enable"=FALSE}}, "EnableStages"=w67, "EnableFIFO"=w66) -> (w65:T7)
    n188 = case shown="True" w202 {
      tunnel: w205 -> [_ w285]
      frame False {
      }
      frame True {
        n189 = xnode "VI-Defined FIFO Configuration"() -> ("FIFO Out"=w280:refnum<k21>)
        n190 = xnode ("FIFO Method Node")("Element"=w285, "Timeout"=0, "FIFO In"=w280) -> ("Timed Out?"=→"NoiseFloorFIFOTimeOut 2":bool)  [unwired: 1 out]
        n191 = call-poly <instrlib>:"Count Up.vi"("increment"=TRUE) -> ("count out"=→"Sends 2":u32)  [unwired: 14 in]
      }
    }
    n192 = Bundle By Name(cluster=w65, "EnableFIFO"=w63) -> (w64:T7)
    n193 = Bundle By Name(cluster=T7 {"EnableFIFO"=FALSE, "EnableStages"={"FreqShiftEnable"=FALSE, "Step4Enable"=FALSE, "Step5Enable"=FALSE, "Step6Enable"=FALSE, "Step7Enable"=FALSE}}, "EnableFIFO"=w58, "EnableStages"="Enable 2") -> (w50:T7)
    n194 = feedback #64() -> (w133:fxp<+/-,48,0>)  [unwired: 1 in]
    n195 = feedback-in #64("FreqShiftCal 2") -> ()
    n196 = feedback #65() -> (w125:T2)  [unwired: 1 in]
    n197 = feedback-in #65("Scale 2") -> ()
    n198 = feedback #66() -> (w131:fxp<+/-,48,0>)  [unwired: 1 in]
    n199 = feedback-in #66("FreqShiftBeac 2") -> ()
    n200 = Bundle By Name(cluster=w50, "EnableFIFO"=w52) -> (w51:T7)
    n201 = call "20210319_Shift_00_ATA_FPGA.vi"("Scale"=w139, "Input valid"=w154, "Index"=w24, "Enable"=w65, "frequency shift"=w135, "Data in"=w218) -> ("Q Shift Output"=w153:T9, "I Shift Output"=w147:T9)  [unwired: 4 in]
    n202 = call "20210319_Shift_00_ATA_FPGA.vi"("Scale"=w125, "Input valid"=w148, "Index"=w24, "Enable"=w50, "frequency shift"=w133, "Data in"=w217) -> ("Q Shift Output"=w49:T9, "I Shift Output"=w57:T9)  [unwired: 4 in]
    n203 = call "20210319_Shift_00_ATA_FPGA.vi"("Scale"=w139, "Input valid"=w154, "Index"=w24, "Enable"=w64, "frequency shift"=w137, "Data in"=w218) -> ("Q Shift Output"=w232:T9, "I Shift Output"=w144:T9)  [unwired: 4 in]
    n204 = call "20210319_Shift_00_ATA_FPGA.vi"("Scale"=w125, "Input valid"=w148, "Index"=w24, "Enable"=w51, "frequency shift"=w131, "Data in"=w217) -> ("Q Shift Output"=w38:T9, "I Shift Output"=w42:T9)  [unwired: 4 in]
    n205 = Unbundle By Name(w147) -> ("output valid"=w79:bool, "Data out"=w72:fxp<+/-,24,1>, "Index"=w74:fxp<+/-,24,1>, "Probe"=w81:T1)
    n206 = Unbundle By Name(w153) -> ("Data out"=w70:fxp<+/-,24,1>, "Index"=w80:fxp<+/-,24,1>, "Probe"=w60:T1)
    n207 = Unbundle By Name(w232) -> ("Data out"=w77:fxp<+/-,24,1>, "Index"=w32:fxp<+/-,24,1>, "Probe"=w76:T1)
    "AI0_Co_Beac_Q_Index" <- w32
    n208 = Unbundle By Name(w57) -> ("output valid"=w56:bool, "Data out"=w55:fxp<+/-,24,1>, "Index"=w54:fxp<+/-,24,1>, "Probe"=w48:T1)
    n209 = Unbundle By Name(w49) -> ("Data out"=w45:fxp<+/-,24,1>, "Index"=w44:fxp<+/-,24,1>, "Probe"=w47:T1)
    n210 = Unbundle By Name(w144) -> ("Probe"=w78:T1, "Data out"=w75:fxp<+/-,24,1>, "Index"=w62:fxp<+/-,24,1>)
    "AI0_Co_I_Index" <- w62
    n211 = Unbundle By Name(w42) -> ("Data out"=w39:fxp<+/-,24,1>, "Index"=w40:fxp<+/-,24,1>, "Probe"=w41:T1)
    n212 = Unbundle By Name(w38) -> ("Data out"=w36:fxp<+/-,24,1>, "Index"=w34:fxp<+/-,24,1>, "Probe"=w37:T1)
    n213 = feedback #67() -> (→"AI0_Cal_IProbe":T1)  [unwired: 1 in]
    n214 = feedback-in #67(w81) -> ()
    n215 = feedback #68() -> (→"Chan0_Cal_QProbe":T1)  [unwired: 1 in]
    n216 = feedback-in #68(w60) -> ()
    n217 = feedback #69() -> (→"Chan0_Beac_IProbe":T1)  [unwired: 1 in]
    n218 = feedback-in #69(w78) -> ()
    n219 = feedback #70() -> (→"Chan0_Beac_QProbe":T1)  [unwired: 1 in]
    n220 = feedback-in #70(w76) -> ()
    n221 = feedback #71() -> (→"Chan1_Cal_IProbe":T1)  [unwired: 1 in]
    n222 = feedback-in #71(w48) -> ()
    n223 = feedback #72() -> (→"Chan1_Cal_QProbe":T1)  [unwired: 1 in]
    n224 = feedback-in #72(w47) -> ()
    n225 = feedback #73() -> (→"Chan1_Beac_IProbe":T1)  [unwired: 1 in]
    n226 = feedback-in #73(w41) -> ()
    n227 = feedback #74() -> (→"Chan1_Beac_QProbe":T1)  [unwired: 1 in]
    n228 = feedback-in #74(w37) -> ()
    n229 = And(x=w79, y="EnableFIFO") -> (x .and. y?=w23:bool)
    "Write to FIFO" <- w23
    n230 = And(x="EnableFIFO", y=w56) -> (x .and. y?=w22:bool)
    n231 = case shown="True" w234 {
      tunnel: w228 -> [_ w308]
      frame False {
      }
      frame True {
        n232 = xnode "VI-Defined FIFO Configuration"() -> ("FIFO Out"=w303:refnum<k21>)
        n233 = xnode ("FIFO Method Node")("Element"=w308, "Timeout"=0, "FIFO In"=w303) -> ("Timed Out?"=→"NoiseFloorFIFOTimeOut":bool)  [unwired: 1 out]
        n234 = call-poly <instrlib>:"Count Up.vi"("increment"=TRUE) -> ("count out"=→"Sends":u32)  [unwired: 14 in]
      }
    }
    n235 = feedback #75() -> (w229:bool)  [unwired: 1 in]
    n236 = feedback-in #75(w23) -> ()
    n237 = feedback #76() -> (w230:fxp<+/-,24,1>)  [unwired: 1 in]
    n238 = feedback-in #76(w72) -> ()
    n239 = feedback #77() -> (w73:fxp<+/-,24,1>)  [unwired: 1 in]
    n240 = feedback-in #77(w74) -> ()
    n241 = feedback #78() -> (w69:fxp<+/-,24,1>)  [unwired: 1 in]
    n242 = feedback-in #78(w70) -> ()
    n243 = feedback #79() -> (w151:fxp<+/-,24,1>)  [unwired: 1 in]
    n244 = feedback-in #79(w80) -> ()
    n245 = feedback #80() -> (w152:fxp<+/-,24,1>)  [unwired: 1 in]
    n246 = feedback-in #80(w75) -> ()
    n247 = feedback #81() -> (w61:fxp<+/-,24,1>)  [unwired: 1 in]
    n248 = feedback-in #81(w62) -> ()
    n249 = feedback #82() -> (w231:fxp<+/-,24,1>)  [unwired: 1 in]
    n250 = feedback-in #82(w77) -> ()
    n251 = feedback #83() -> (w71:fxp<+/-,24,1>)  [unwired: 1 in]
    n252 = feedback-in #83(w32) -> ()
    n253 = feedback #84() -> (w20:bool)  [unwired: 1 in]
    "Write to FIFO 2" <- w20
    n254 = feedback-in #84(w22) -> ()
    n255 = feedback #85() -> (w204:fxp<+/-,24,1>)  [unwired: 1 in]
    n256 = feedback-in #85(w55) -> ()
    n257 = feedback #86() -> (w46:fxp<+/-,24,1>)  [unwired: 1 in]
    n258 = feedback-in #86(w54) -> ()
    n259 = feedback #87() -> (w149:fxp<+/-,24,1>)  [unwired: 1 in]
    n260 = feedback-in #87(w45) -> ()
    n261 = feedback #88() -> (w43:fxp<+/-,24,1>)  [unwired: 1 in]
    n262 = feedback-in #88(w44) -> ()
    n263 = feedback #89() -> (w150:fxp<+/-,24,1>)  [unwired: 1 in]
    n264 = feedback-in #89(w39) -> ()
    n265 = feedback #90() -> (w203:fxp<+/-,24,1>)  [unwired: 1 in]
    n266 = feedback-in #90(w40) -> ()
    n267 = feedback #91() -> (w35:fxp<+/-,24,1>)  [unwired: 1 in]
    n268 = feedback-in #91(w36) -> ()
    n269 = feedback #92() -> (w33:fxp<+/-,24,1>)  [unwired: 1 in]
    n270 = feedback-in #92(w34) -> ()
    n271 = case shown="True" w229 {
      tunnel: w230 -> [_ w322]
      tunnel: w231 -> [_ w311]
      tunnel: w152 -> [_ w309]
      tunnel: w151 -> [_ w317]
      tunnel: w73 -> [_ w320]
      tunnel: w69 -> [_ w318]
      tunnel: w71 -> [_ w319]
      tunnel: w61 -> [_ w316]
      frame False {
        # "Ready last time?"
      }
      frame True {
        # "Ramp function can be enabled\nfor test/debug"
        # "Transfer when data is valid.\nMost of the time the data is NOT\nvalid as a result of drastic decimation"
        n272 = call-poly <instrlib>:"Count Up.vi"("increment"=TRUE) -> ("count out"=w324:u32)  [unwired: 14 in]
        n273 = To Fixed-Point(fixed-point type=fxp<+/-,24,1> 0.0, number=w324) -> (fixed-point=w323:fxp<+/-,24,1>)
        n274 = feedback-in #93(w323) -> ()
        n275 = feedback #93() -> (w313:fxp<+/-,24,1>)  [unwired: 1 in]
        n276 = Select(t=w313, s="Ramp?", f=w322) -> (s? t:f=w321:fxp<+/-,24,1>)
        n277 = Select(t=w313, s="Ramp?", f=w309) -> (s? t:f=w310:fxp<+/-,24,1>)
        n278 = Build Array(w321, w320, w318, w317, w310, w316, w311, w319) -> (w315:fxp<+/-,24,1>[])
        n279 = xnode ("FIFO Method Node")("Element"=w315, "Timeout"=0) -> ()  [unwired: 1 in, 2 out]
      }
    }
    n280 = case shown="True" w20 {
      tunnel: w204 -> [_ w301]
      tunnel: w203 -> [_ w297]
      tunnel: w150 -> [_ w289]
      tunnel: w149 -> [_ w299]
      tunnel: w46 -> [_ w300]
      tunnel: w43 -> [_ w298]
      tunnel: w35 -> [_ w296]
      tunnel: w33 -> [_ w295]
      frame False {
      }
      frame True {
        # "Ramp function can be enabled\nfor test/debug"
        # "Transfer when data is valid.\nMost of the time the data is NOT\nvalid as a result of drastic decimation"
        n281 = call-poly <instrlib>:"Count Up.vi"("increment"=TRUE) -> ("count out"=w292:u32)  [unwired: 14 in]
        n282 = To Fixed-Point(fixed-point type=fxp<+/-,24,1> 0.0, number=w292) -> (fixed-point=w291:fxp<+/-,24,1>)
        n283 = local read "Ramp?"() -> (w287:bool)
        n284 = feedback #94() -> (w290:fxp<+/-,24,1>)  [unwired: 1 in]
        n285 = feedback-in #94(w291) -> ()
        n286 = Select(t=w290, s=w287, f=w289) -> (s? t:f=w288:fxp<+/-,24,1>)
        n287 = Build Array(w301, w300, w299, w298, w288, w297, w296, w295) -> (w302:fxp<+/-,24,1>[])
        n288 = xnode ("FIFO Method Node")("Element"=w302, "Timeout"=0) -> ()  [unwired: 1 in, 2 out]
      }
    }
  }
  n289 = while {
    stop <- FALSE stop-if-true
    # "Initialization Done:\nThis node will be true when the Adapter Module has finished configuring itself and is generating valid samples."
    # "Configuration Loop"
    n290 = xnode "FPGA I/O Node"() -> ("IO Module\\Initialization Done"=→"IO Module\\Initialization Done")  [unwired: 1 in, 1 out]
  }
  n291 = while {
    stop <- FALSE stop-if-true
    # "Clock Commit has a built in rising edge detector. Refer to the NI 5762 Component-Level IP Reference section of the LabVIEW FPGA Module Help for more information."
    # "This loop configures the Sample clock selection for the NI 5762. Refer to the Clock Select (Host).vi Host VI for more information about how this example configures the clock."
    n292 = xnode "FPGA I/O Node"("IO Module\\Sample Clock Select"="Sample Clock Select", "IO Module\\Sample Clock Commit"="Sample Clock Commit") -> ("IO Module\\SPI Idle"=→"SPI Idle", "IO Module\\Configuration Error"=→"Configuration Error", "IO Module\\PLL Locked"=→"Synthesizer Locked")  [unwired: 5 in, 5 out]
  }
  n293 = xnode "VI-Defined Memory"() -> ("Memory Out"=w7:refnum<k21>)
  n294 = xnode "VI-Defined Memory"() -> ("Memory Out"=w6:refnum<k21>)
  n295 = for {
    N: 8192 ("dimension size") -> [_]
    tunnel: [w338] -> w8
    tunnel: w7 -> [w337]
    i -> [w341]
    n296 = To Unsigned Long Integer(number=w341) -> (unsigned 32bit integer=w340:u32)
    n297 = xnode ("Memory Method Node")("Address"=w340, "Data"=fxp<+/-,27,12> 0.0, "Memory In"=w337) -> ("Memory Out"=w338:refnum<k21>)
  }
  n298 = for {
    N: 8192 ("dimension size") -> [_]
    tunnel: [w343] -> w5
    tunnel: w6 -> [w342]
    i -> [w346]
    n299 = To Unsigned Long Integer(number=w346) -> (unsigned 32bit integer=w345:u32)
    n300 = xnode ("Memory Method Node")("Address"=w345, "Data"=fxp<+/-,27,12> 0.0, "Memory In"=w342) -> ("Memory Out"=w343:refnum<k21>)
  }
  n301 = while {
    shift-right: [w349] -> _
    shift-left: TRUE -> [w350]
    tunnel: w8 -> [w347]
    i -> [w351]
    stop <- FALSE stop-if-true
    # "Most recent processed point"
    # "Noise Floor FFT"
    n302 = xnode ("FIFO Method Node")("Timeout"=0) -> ("Element"=w353:fxp<+/-,16,1>, "Timed Out?"=w348:bool)  [unwired: 1 in, 1 out]
    "ReceiverTimed Out" <- w348
    n303 = case shown="False" w348 {
      tunnel: w353 -> [w380 _]
      tunnel: w350 -> [w379 w412]
      tunnel: [FALSE w412] -> w349
      tunnel: w347 -> [w361 _]
      frame False {
        # "Squaring FFT values so we can add them. \nOtherwise we get destructive interference and the averaging doesn't work."
        # "Must be greater/equal.\nEqual can get stuck if the user\ndecreases #Avg value.\n3-14-2019"
        # "Is collection of frames finished?"
        # "Is frame finished?"
        # "Build sum of many FFT frames, point by point."
        n304 = xnode ("FFT")("real data in"=w380, "reset"=w379, "imaginary data in"=fxp<+/-,16,1> 0.0) -> ("data index"=w372:u16, "real data out"=w358:fxp<+/-,30,15>)  [unwired: 1 out]
        n305 = To Unsigned Long Integer(number=w372) -> (unsigned 32bit integer=w364:u32)
        n306 = xnode ("Memory Method Node")("Address"=w364, "Memory In"=w361) -> ("Data"=w363:fxp<+/-,27,12>, "Memory Out"=w360:refnum<k21>)
        n307 = feedback #95() -> (w374:u16)  [unwired: 1 in]
        n308 = feedback-in #95(w372) -> ()
        n309 = xnode ("High Throughput Multiply")("x"=w358, "y"=w358) -> ("x*y"=w357:fxp<+/-,60,30>)
        n310 = Build Array(w372, w374) -> (→"SuccessiveIndeces":u16[])
        n311 = To Fixed-Point(fixed-point type=fxp<+/-,27,12> 0.0 ("Data"), number=w357) -> (fixed-point=w355:fxp<+/-,27,12>)
        n312 = xnode ("High Throughput Add")("x"=w363, "y"=w355) -> ("x+y"=w362:fxp<+/-,28,13>)  [unwired: 1 out]
        n313 = To Fixed-Point(fixed-point type=fxp<+/-,27,12> 0.0 ("Data"), number=w362) -> (fixed-point=w365:fxp<+/-,27,12>)
        n314 = Greater Or Equal?(x=w372, y=u16 8191) -> (x >= y?=w367:bool)
        n315 = xnode ("Memory Method Node")("Address"=w364, "Data"=w365, "Memory In"=w360) -> ("Memory Out"=w359:refnum<k21>)
        n316 = feedback #96(FALSE) -> (w370:bool)
        n317 = call-poly <instrlib>:"Count Up.vi"("increment"=w367, "reset"=w370) -> ("count out"=w369:u16)  [unwired: 13 in]
        n318 = Greater Or Equal?(x=w369, y="#Avg") -> (x >= y?=w377:bool)
        n319 = feedback-in #96(w377) -> ()
        n320 = case shown="True" w377 {
          tunnel: w359 -> [_ w400]
          frame False {
          }
          frame True {
            n321 = for {
              N: 8192 ("dimension size") -> [_]
              tunnel: w400 -> [w402]
              i -> [w405]
              # "Transfer summed collection of frames to host."
              # "Reset to zeros"
              n322 = To Unsigned Long Integer(number=w405) -> (unsigned 32bit integer=w407:u32)
              n323 = xnode ("Memory Method Node")("Address"=w407, "Memory In"=w402) -> ("Data"=w406:fxp<+/-,27,12>, "Memory Out"=w403:refnum<k21>)
              n324 = Integer to Fixed-Point Cast(fixed-point type=fxp<+/-,30,15> 0.0 ("real data out"), integer=w405) -> (fixed-point=w410:fxp<+/-,30,15>)
              n325 = Build Array(w410, w406) -> (w408:fxp<+/-,30,15>[])
              n326 = xnode ("Memory Method Node")("Address"=w407, "Data"=fxp<+/-,27,12> 0.0, "Memory In"=w403) -> ()  [unwired: 1 out]
              n327 = xnode ("FIFO Method Node")("Element"=w408, "Timeout"=0) -> ()  [unwired: 1 in, 2 out]
            }
          }
        }
      }
      frame True {
      }
    }
    "NoiseFloorFFT_LoopCount" <- w351
  }
  n328 = while {
    shift-right: [w415] -> _
    shift-left: TRUE -> [w416]
    tunnel: w5 -> [w413]
    i -> [w417]
    stop <- FALSE stop-if-true
    # "Most recent processed point"
    # "Noise Floor FFT"
    n329 = xnode ("FIFO Method Node")("Timeout"=0) -> ("Element"=w419:fxp<+/-,16,1>, "Timed Out?"=w414:bool)  [unwired: 1 in, 1 out]
    "ReceiverTimed Out 2" <- w414
    n330 = case shown="False" w414 {
      tunnel: w419 -> [w446 _]
      tunnel: w416 -> [w445 w478]
      tunnel: [FALSE w478] -> w415
      tunnel: w413 -> [w427 _]
      frame False {
        # "Is collection of frames finished?"
        # "Is frame finished?"
        # "Build sum of many FFT frames, point by point."
        n331 = xnode ("FFT 2")("real data in"=w446, "reset"=w445, "imaginary data in"=fxp<+/-,16,1> 0.0) -> ("data index"=w438:u16, "real data out"=w422:fxp<+/-,30,15>)  [unwired: 1 out]
        n332 = To Unsigned Long Integer(number=w438) -> (unsigned 32bit integer=w430:u32)
        n333 = xnode ("Memory Method Node")("Address"=w430, "Memory In"=w427) -> ("Data"=w429:fxp<+/-,27,12>, "Memory Out"=w426:refnum<k21>)
        n334 = feedback #97() -> (w440:u16)  [unwired: 1 in]
        n335 = feedback-in #97(w438) -> ()
        n336 = xnode ("High Throughput Multiply")("x"=w422, "y"=w422) -> ("x*y"=w424:fxp<+/-,60,30>)
        n337 = Build Array(w438, w440) -> (→"SuccessiveIndeces 2":u16[])
        n338 = To Fixed-Point(fixed-point type=fxp<+/-,27,12> 0.0 ("Data"), number=w424) -> (fixed-point=w421:fxp<+/-,27,12>)
        n339 = xnode ("High Throughput Add")("x"=w429, "y"=w421) -> ("x+y"=w428:fxp<+/-,28,13>)  [unwired: 1 out]
        n340 = To Fixed-Point(fixed-point type=fxp<+/-,27,12> 0.0 ("Data"), number=w428) -> (fixed-point=w431:fxp<+/-,27,12>)
        n341 = Greater Or Equal?(x=w438, y=u16 8191) -> (x >= y?=w433:bool)
        n342 = xnode ("Memory Method Node")("Address"=w430, "Data"=w431, "Memory In"=w426) -> ("Memory Out"=w425:refnum<k21>)
        n343 = feedback #98(FALSE) -> (w436:bool)
        n344 = call-poly <instrlib>:"Count Up.vi"("increment"=w433, "reset"=w436) -> ("count out"=w435:u16)  [unwired: 13 in]
        n345 = Greater Or Equal?(x=w435, y="#Avg 2") -> (x >= y?=w443:bool)
        n346 = feedback-in #98(w443) -> ()
        n347 = case shown="True" w443 {
          tunnel: w425 -> [_ w466]
          frame False {
          }
          frame True {
            n348 = for {
              N: 8192 ("dimension size") -> [_]
              tunnel: w466 -> [w468]
              i -> [w471]
              # "Transfer summed collection of frames to host."
              # "Reset to zeros"
              n349 = To Unsigned Long Integer(number=w471) -> (unsigned 32bit integer=w473:u32)
              n350 = xnode ("Memory Method Node")("Address"=w473, "Memory In"=w468) -> ("Data"=w472:fxp<+/-,27,12>, "Memory Out"=w469:refnum<k21>)
              n351 = Integer to Fixed-Point Cast(fixed-point type=fxp<+/-,30,15> 0.0 ("real data out"), integer=w471) -> (fixed-point=w476:fxp<+/-,30,15>)
              n352 = Build Array(w476, w472) -> (w474:fxp<+/-,30,15>[])
              n353 = xnode ("Memory Method Node")("Address"=w473, "Data"=fxp<+/-,27,12> 0.0, "Memory In"=w469) -> ()  [unwired: 1 out]
              n354 = xnode ("FIFO Method Node")("Element"=w474, "Timeout"=0) -> ()  [unwired: 1 in, 2 out]
            }
          }
        }
      }
      frame True {
      }
    }
    "NoiseFloorFFT_LoopCount 2" <- w417
  }
  n355 = node-c288(w12) -> ()
